vi "FTW-Test-EndpointListener.vi"() -> (0 "error out":errorcluster)   [LabVIEW 2013]
uses:
  source/actor/Ether/FTW-Ether-EndpointType.ctl
  source/actor/Payload/FTW-MessagePayload.ctl
  source/actor/Endpoint/FTW-Endpoint.lvclass
  source/actor/Ether/FTW-Ether.lvclass
panel:
  in  "Connection":string(combo)="tcp://127.0.0.1:62023"
  out "Timed out?":bool
  out "Actual Server Address":string
  out "Response Body":string
  out "Response Header":string
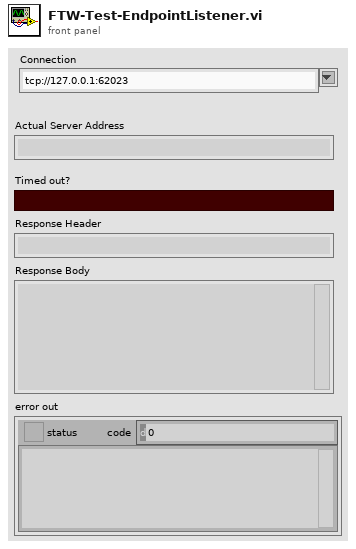
[diagram p1: front panel]
types:
  T1 = typedef "FTW-MessagePayload.ctl" = cluster{"Header":string, "Body":string, "Metadata":string}
  T2 = typedef "FTW-Ether.lvclass/FTW-Ether-EndpointType.ctl" = enum16{"Server", "Client", "Publisher", "Subscriber"}
  T3 = typedef "FTW-Ether.lvclass/FTW-Ether-MessageTransportScheme.ctl" = enum16{"In process (inproc://)", "TCP (tcp://)"}
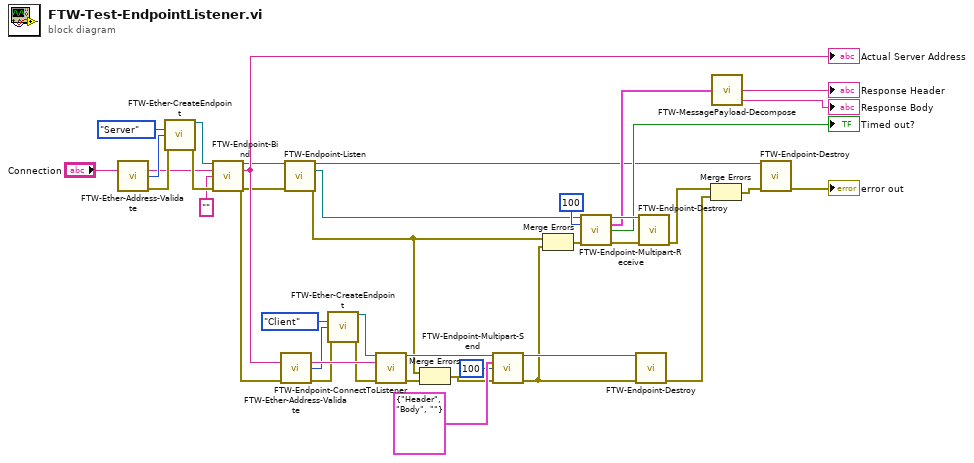
[diagram p0: block diagram]
diagram:
  n1 = call "FTW-Ether-Address-Validate.vi"("Address"="Connection") -> ("Sanitized Address"=w17:string, "Message Transport Scheme"=w22:T3, "error out"=w19:errorcluster)  [unwired: 12 in]
  n2 = call "FTW-Ether-CreateEndpoint.vi"("Endpoint Type"=FTW-Ether-EndpointType."Server", "Message Transport Scheme"=w22, "error in"=w19) -> ("FTW Endpoint"=w21:refnum<class "FTW-Endpoint.lvclass">, "error out"=w20:errorcluster)  [unwired: 11 in]
  n3 = call-dynamic "FTW-Endpoint-Bind.vi"("FTW Endpoint"=w21, "Endpoint Address"=w17, "Requested Identity"="", "error in"=w20) -> ("FTW Endpoint out"=w10:refnum<class "FTW-Endpoint.lvclass">, "Actual Endpoint Address"=w15:string, "error out"=w9:errorcluster)  [unwired: 8 in, 1 out]
  "Actual Server Address" <- w15
  n4 = call "FTW-Ether-Address-Validate.vi"("Address"=w15, "error in"=w9) -> ("Sanitized Address"=w29:string, "Message Transport Scheme"=w25:T3, "error out"=w28:errorcluster)  [unwired: 11 in]
  n5 = call-dynamic "FTW-Endpoint-Listen.vi"("FTW Endpoint"=w10, "error in"=w9) -> ("FTW Endpoint out"=w6:refnum<class "FTW-Endpoint.lvclass">, "New Connection"=w8:refnum<class "FTW-Endpoint.lvclass">, "error out"=w1:errorcluster)  [unwired: 11 in]
  n6 = call "FTW-Ether-CreateEndpoint.vi"("Endpoint Type"=FTW-Ether-EndpointType."Client", "Message Transport Scheme"=w25, "error in"=w28) -> ("FTW Endpoint"=w26:refnum<class "FTW-Endpoint.lvclass">, "error out"=w27:errorcluster)  [unwired: 11 in]
  n7 = call-dynamic "FTW-Endpoint-ConnectToListener.vi"("FTW-Endpoint In"=w26, "Address"=w29, "error in"=w27) -> ("FTW-Endpoint Out"=w39:refnum<class "FTW-Endpoint.lvclass">, "error out"=w5:errorcluster)  [unwired: 10 in, 1 out]
  n8 = Merge Errors(w1, w5) -> (w2:errorcluster)
  n9 = call-dynamic "FTW-Endpoint-Multipart-Send.vi"("FTW Endpoint"=w39, "Message"=T1 {"Header"="Header", "Body"="Body", "Metadata"=""}, "Timeout"=100, "error in"=w2) -> ("FTW Endpoint out"=w38:refnum<class "FTW-Endpoint.lvclass">, "error out"=w3:errorcluster)  [unwired: 9 in, 1 out]
  n10 = Merge Errors(w1, w3) -> (w4:errorcluster)
  n11 = call-dynamic "FTW-Endpoint-Multipart-Receive.vi"("FTW Endpoint"=w8, "Timeout"=100, "error in"=w4) -> ("FTW Endpoint out"=w37:refnum<class "FTW-Endpoint.lvclass">, "Message Received"=w35:T1, "Timed out?"=→"Timed out?":bool, "error out"=w36:errorcluster)  [unwired: 9 in]
  n12 = call-dynamic "FTW-Endpoint-Destroy.vi"("FTW Endpoint"=w38, "error in"=w3) -> ("error out"=w33:errorcluster)  [unwired: 13 in]
  n13 = call-dynamic "FTW-Endpoint-Destroy.vi"("FTW Endpoint"=w37, "error in"=w36) -> ("error out"=w34:errorcluster)  [unwired: 13 in]
  n14 = Merge Errors(w34, w33) -> (w32:errorcluster)
  n15 = call "FTW-MessagePayload-Decompose.vi"("Message"=w35) -> ("Message Header"=→"Response Header":string, "Message Body"=→"Response Body":string)  [unwired: 1 in, 1 out]
  n16 = call-dynamic "FTW-Endpoint-Destroy.vi"("FTW Endpoint"=w6, "error in"=w32) -> ("error out"=→"error out":errorcluster)  [unwired: 13 in]
